vi "Three devices.vi"() -> ()   [LabVIEW 2015]
doc: "This example VI shows how to convert string data elements to numeric elements so it can be graphed and displayed on an XY Graph."
uses:
  <instrlib>/Keithley 27XX/Public/Configure/Measurement Specific/Configure Thermocouple.vi
  <instrlib>/Ke24xx/Ke24xx.llb/Ke24xx Configure Source Volt/Cur Level.vi
  <instrlib>/Ke24xx/Ke24xx.llb/Ke24xx Enable/Disable Source Output.vi
  <instrlib>/Keithley 27XX/Keithley 27XX.lvlib
panel:
  in  "Compliance":dbl=1.0 min=-1100.0 max=1100.0 step=1.0 format="%.2p"
  out "error out Cryocon":errorcluster
  out "error out 2425":errorcluster
  in  "Loop 2":bool
  in  "level":dbl=12.0 min=-1100.0 max=1100.0 step=1.0 format="%.2p"
  in  "range":i32
  in  "function":i32(slide)
  in  "error in (no error) 2":errorcluster
  in  "reset device":u16(slide)=1
  in  "id query":u16(slide)=1
  in  "resource name":string="GPIB0::20::INSTR"
  out "Delta":dbl
  out "Variance":string
  in  "Setpoint":dbl=300.0
  in  "D":sgl format="%.2f"
  in  "I":sgl=30.0 min=0 step=1 format="%.2f"
  in  "P":sgl=5.0 format="%.2f"
  in  "Output":u8(ring) items=["Loop 1", "Loop 2"]
  in  "Loop 1":bool
  out "Minimum":string
  out "Time Since Reset (Mins)":string
  out "Maximum":string
  out "Offset":string
  out "Cryocon Temp":dbl(graph)
  in  "Set Input":u8(ring) items=["ChA", "ChB", "ChC", "ChD"]
  in  "error in (no error)":errorcluster
  in  "baud rate (9600)":u32=9600
  in  "Port":string="10::INSTR"
  in  "Interface":u16(ring) items=["GPIB", "Serial"]
  in  "Save File?":bool
  out "Channel 3":dbl[](graph)
  out "Channel 2":dbl[](graph)
  out "Channel 1":dbl[](graph)
  in  "Enable Open Detector? (False)":bool
  in  "Simulated Reference Temperature (23 deg C)":dbl=23.0
  in  "Reference Junction Type (0: Simulated)":u16(ring)=1 items=["Simulated", "Internal", "External"]
  in  "Thermocouple Type (1: K)":u16(ring)=1 items=["J", "K", "T", "E", "R", "S", "B", "N"]
  in  "Column headers":string[](array[string])=["Time/s", "Cryocon Temp/C", "Ch101 Temp/C", "", "", "", ""]
  in  "Number of channels":i32=1
  in  "Pause/Continue":bool
  in  "stop":bool
  out "Iterations":i32
  out "concatenated string":string
  in  "file (use dialog)":path=path "C:/Users/Guest_2/Desktop/Zong Long/Data trial.txt"
  in  "Function (6: Temp)":u16(ring)=6 items=["DC Voltage", "AC Voltage", "DC Current", "AC Current", "Resistance", "Four-Wire Resistance", "Temperature (C)", "Frequency", "Period", "Continuity"]
  in  "Channel List (101)":string="101"
  in  "Serial Configuration":T1={"Baud Rate (9600)"=9600, "Flow Control (1: XON/XOFF)"=1, "Termination Char (0:CR)"=0} {"Termination Char (0:CR)" items=["CR", "LF", "CRLF (Do not use)", "LFCR (Do not use)"]; "Flow Control (1: XON/XOFF)" items=["None", "XON/XOFF", "RTS/CTS (2701 Only)", "XON/XOFF & RTS/CTS (2701 Only)"]; "Baud Rate (9600)" items=["300"=300, "600"=600, "1200"=1200, "2400"=2400, "4800"=4800, "9600"=9600, "19.2k"=19200, "38.4k (2701 Only)"=38400, "57.6k (2701 Only)"=57600, "115.2k (2701 Only)"=115200]}
  in  "Keithley VISA \nresource name":refnum<visa-resource-name>="GPIB0::19::INSTR"
  # "Keithley 2425 INIT"
  # "Cryocon INIT"
  # "File INIT"
  # "Keithley 2700 INIT"
  # "Operations"
  # "Data"
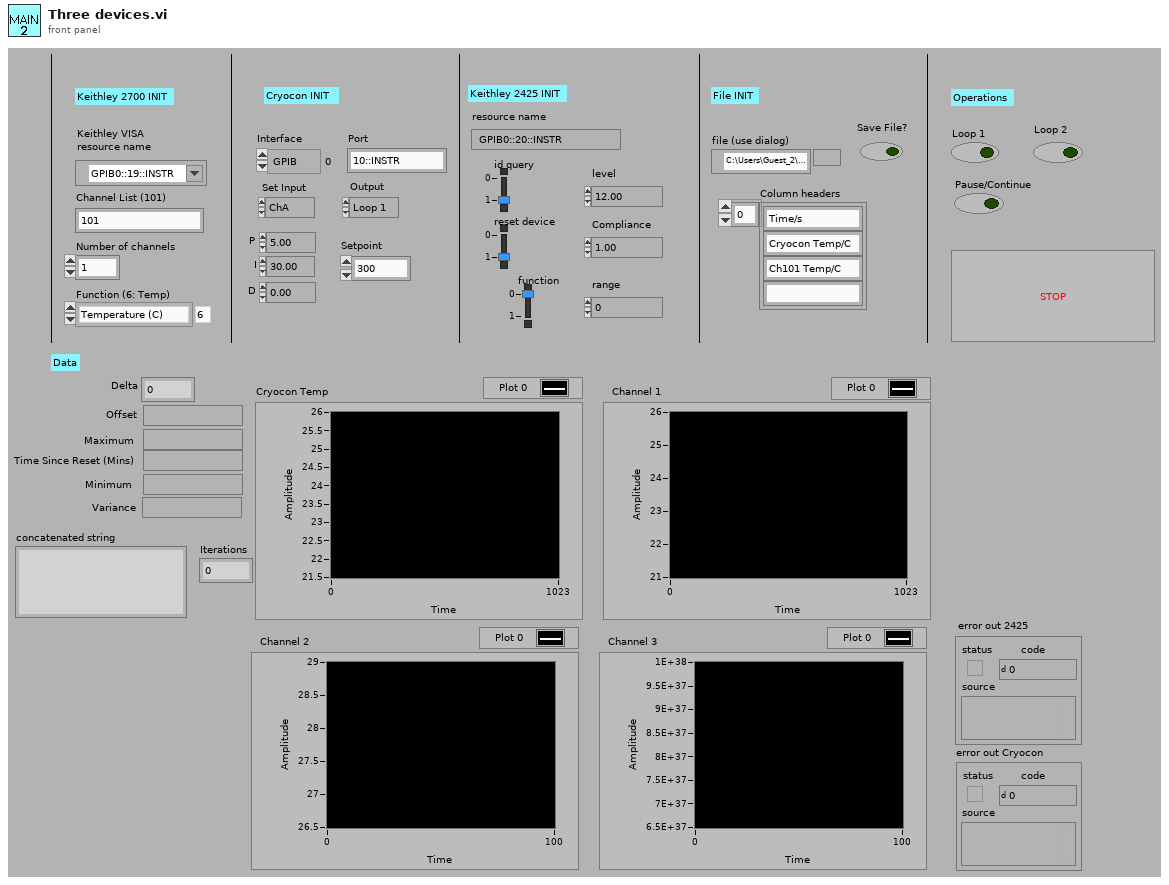
[diagram p1: front panel]
types:
  T1 = cluster{"Baud Rate (9600)":u32, "Flow Control (1: XON/XOFF)":u16, "Termination Char (0:CR)":u16}
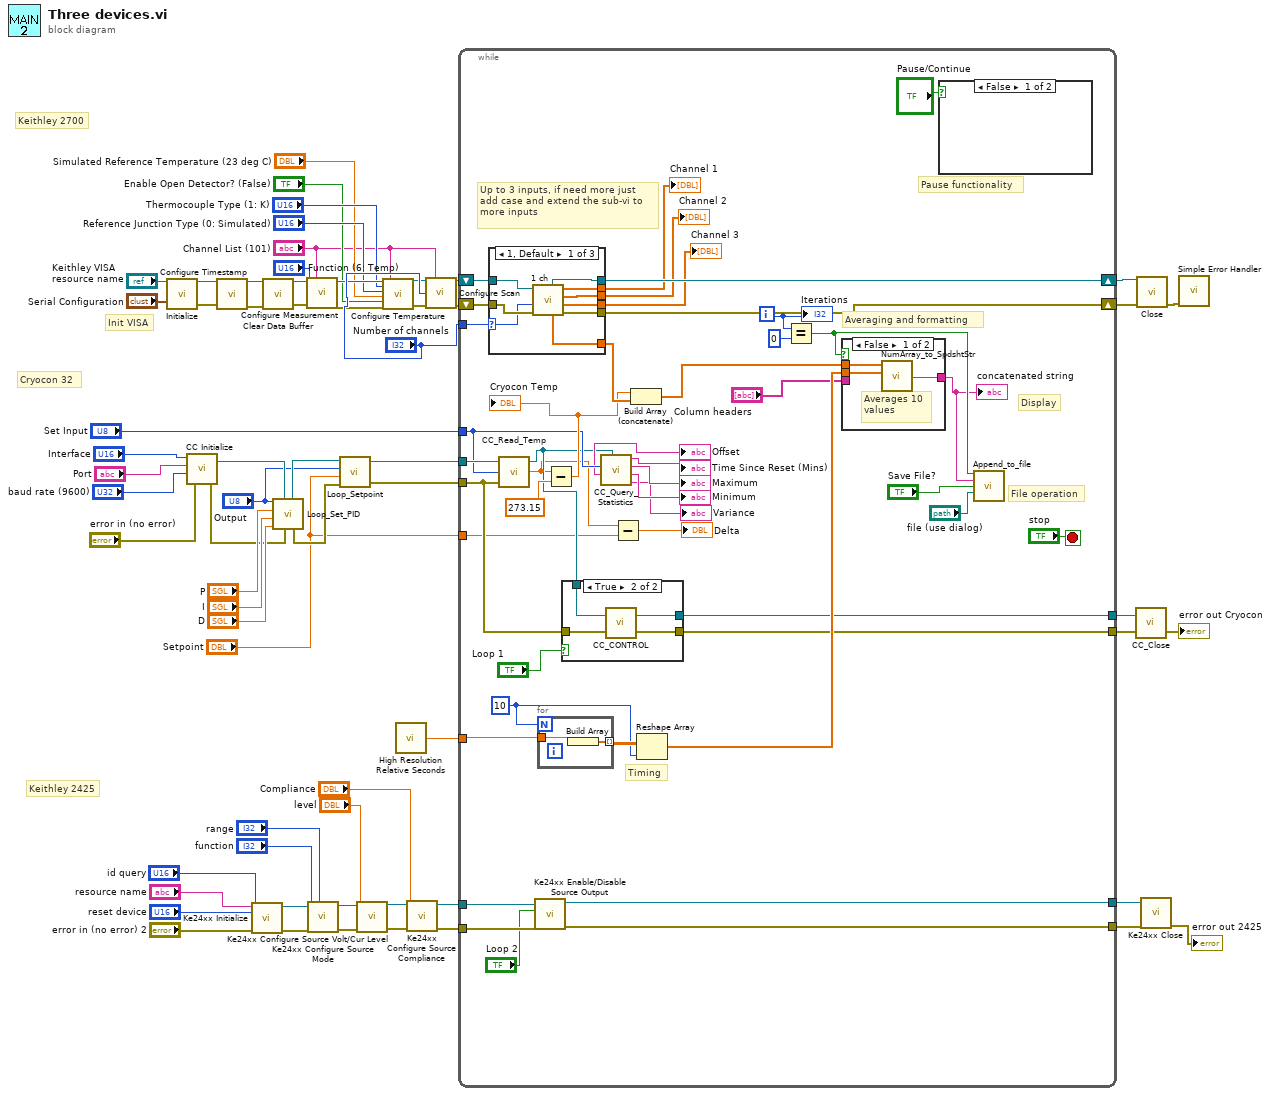
[diagram p0: block diagram]
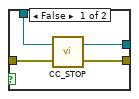
[diagram p2: hidden frame]
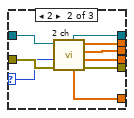
[diagram p3: hidden frame]
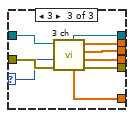
[diagram p4: hidden frame]
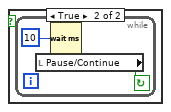
[diagram p5: hidden frame]
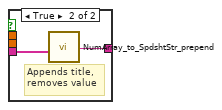
[diagram p6: hidden frame]
diagram:
  # "Keithley 2425"
  # "Cryocon 32"
  # "Keithley 2700"
  # "Init VISA"
  n1 = call <instrlib>:"Initialize.vi"("VISA resource name"="Keithley VISA \nresource name", "Serial Configuration"="Serial Configuration") -> ("VISA resource name out"=w60:refnum<visa-resource-name>, "error out"=w59:errorcluster)  [unwired: 12 in]
  n2 = call "CC Initialize.vi"("error in (no error)"="error in (no error)", "baud rate (9600)"="baud rate (9600)", "Port"="Port", "Interface"="Interface") -> ("error out"=w28:errorcluster, "VISA out"=w27:refnum<visa-resource-name>)
  n3 = call <instrlib>:"Configure Timestamp.vi"("VISA resource name"=w60, "error in (no error)"=w59) -> ("VISA resource name out"=w55:refnum<visa-resource-name>, "error out"=w54:errorcluster)  [unwired: 12 in]
  n4 = call <instrlib>:"Ke24xx Initialize.vi"("error in (no error)"="error in (no error) 2", "reset device"="reset device", "id query"="id query", "resource name"="resource name") -> ("error out"=w15:errorcluster, "instrument handle out"=w16:refnum<visa-resource-name>)  [unwired: 5 in, 1 out]
  n5 = call <instrlib>:"Clear Data Buffer.vi"("VISA resource name"=w55, "error in (no error)"=w54) -> ("VISA resource name out"=w53:refnum<visa-resource-name>, "error out"=w56:errorcluster)  [unwired: 12 in]
  n6 = call "Loop_Set_PID"("error in (no error)"=w28, "VISA In"=w27, "D"="D", "I"="I", "P"="P", "Output"="Output") -> ("error out"=w26:errorcluster, "VISA Out"=w25:refnum<visa-resource-name>)  [unwired: 4 in]
  n7 = call <instrlib>:"Configure Measurement.vi"("VISA resource name"=w53, "Scan List (Empty)"="Channel List (101)", "Function (0: DC Voltage)"="Function (6: Temp)", "error in (no error)"=w56) -> ("VISA resource name out"=w47:refnum<visa-resource-name>, "error out"=w44:errorcluster)  [unwired: 10 in]
  n8 = call <instrlib>:"Ke24xx Configure Source Mode.vi"("range"="range", "error in (no error)"=w15, "function"="function", "instrument handle"=w16) -> ("error out"=w11:errorcluster, "instrument handle out"=w12:refnum<visa-resource-name>)  [unwired: 5 in, 1 out]
  n9 = call "Loop_Setpoint.vi"("VISA in"=w25, "Loop"="Output", "Setpoint"="Setpoint", "error in"=w26) -> ("VISA out"=w24:refnum<visa-resource-name>, "ErrorOut"=w22:errorcluster)  [unwired: 1 in, 1 out]
  n10 = call "Ke24xx Configure Source Volt/Cur Level.vi"("error in (no error)"=w11, "level"="level", "instrument handle"=w12) -> ("error out"=w10:errorcluster, "instrument handle out"=w9:refnum<visa-resource-name>)  [unwired: 6 in, 1 out]
  n11 = call-poly <instrlib>:"Configure Temperature.vi"("VISA resource name"=w47, "Thermocouple Type (1: K)"="Thermocouple Type (1: K)", "Reference Junction Type (0: Simulated)"="Reference Junction Type (0: Simulated)", "Simulated Reference Temperature (23 deg C)"="Simulated Reference Temperature (23 deg C)", "Enable Open Detector? (False)"="Enable Open Detector? (False)", "error in (no error)"=w44, "Scan List (Empty)"="Channel List (101)") -> ("VISA resource name out"=w46:refnum<visa-resource-name>, "error out"=w45:errorcluster)  [unwired: 11 in]
  n12 = call <vilib>:"High Resolution Relative Seconds.vi"() -> ("relative seconds"=w49:dbl)
  n13 = call <instrlib>:"Ke24xx Configure Source Compliance.vi"("error in (no error)"=w10, "level"="Compliance", "instrument handle"=w9) -> ("error out"=w6:errorcluster, "instrument handle out"=w7:refnum<visa-resource-name>)  [unwired: 6 in, 1 out]
  n14 = call <instrlib>:"Configure Scan.vi"("VISA resource name"=w46, "Channel List (101:110)"="Channel List (101)", "Sample Count (100)"="Number of channels", "error in (no error)"=w45) -> ("VISA resource name out"=w51:refnum<visa-resource-name>, "error out"=w50:errorcluster)  [unwired: 10 in]
  n15 = while {
    shift-right: [w107] -> w57
    shift-left: w51 -> [w106]
    shift-right: [w108] -> w58
    shift-left: w50 -> [w105]
    tunnel: w49 -> [w103]
    tunnel: "Number of channels" -> [w96]
    tunnel: "Set Input" -> [w82]
    tunnel: w24 -> [w87]
    tunnel: w22 -> [w75]
    tunnel: [w74] -> w33
    tunnel: [w73] -> w32
    tunnel: "Setpoint" -> [w70]
    tunnel: w7 -> [w68]
    tunnel: w6 -> [w67]
    tunnel: [w65] -> w5
    tunnel: [w64] -> w4
    i -> [w98]
    stop <- "stop" stop-if-true
    w95 = 10 ("x")
    # "Timing"
    # "Up to 3 inputs, if need more just\nadd case and extend the sub-vi to\nmore inputs"
    # "Display"
    # "Averaging and formatting"
    # "File operation"
    # "Pause functionality"
    n16 = case shown="1, Default" w96 {
      selector: w96 -> [w124 w131 w140]
      tunnel: [w120 w132 w141] -> w108
      tunnel: [w122 w129 w139] -> w107
      tunnel: w106 -> [w123 w134 w142]
      tunnel: w105 -> [w125 w133 w143]
      tunnel: [w119 w127 w137] -> w92
      tunnel: [w118 w128 w136] -> w94
      tunnel: [w117 w130 w135] -> w93
      tunnel: [w121 w126 w138] -> w85
      frame 1, Default {
        n17 = call "1 ch.vi"("error out"=w125, "Number of channels"=w124, "VISA resource name out"=w123) -> ("error out 2"=w120:errorcluster, "output array 3"=w117:dbl[], "output array 2"=w118:dbl[], "Means of 10"=w119:dbl[], "output array"=w121:dbl[], "VISA resource name out 2"=w122:refnum<visa-resource-name>)  [unwired: 3 in]
      }
      frame 2 {
        n18 = call "2 ch.vi"("error out"=w133, "Number of channels"=w131, "VISA resource name out"=w134) -> ("error out 2"=w132:errorcluster, "Means of 12"=w130:dbl[], "Means of 11"=w128:dbl[], "Means of 10"=w127:dbl[], "output array"=w126:dbl[], "VISA resource name out 2"=w129:refnum<visa-resource-name>)  [unwired: 3 in]
      }
      frame 3 {
        n19 = call "3 ch.vi"("error out"=w143, "Number of channels"=w140, "VISA resource name out"=w142) -> ("error out 2"=w141:errorcluster, "Means of 12"=w135:dbl[], "Means of 11"=w136:dbl[], "Means of 10"=w137:dbl[], "output array"=w138:dbl[], "VISA resource name out 2"=w139:refnum<visa-resource-name>)  [unwired: 3 in]
      }
    }
    "Channel 3" <- w93
    "Channel 2" <- w94
    "Channel 1" <- w92
    n20 = call "CC_Read_Temp.vi"("error in (no error)"=w75, "Input"=w82, "VISA In"=w87) -> ("Temperature"=w71:dbl, "VISA Out"=w76:refnum<visa-resource-name>)  [unwired: 1 out]
    n21 = call "Ke24xx Enable/Disable Source Output.vi"("error in (no error)"=w67, "state"="Loop 2", "instrument handle"=w68) -> ("error out"=w64:errorcluster, "instrument handle out"=w65:refnum<visa-resource-name>)  [unwired: 6 in, 1 out]
    n22 = for {
      N: w95 -> [_]
      tunnel: w103 -> [w147]
      tunnel: [w146] -> w102 mode=indexing
      n23 = Build Array(w147) -> (w146:dbl[])
    }
    n24 = Subtract(x=w71, y=273.15) -> (x-y=w83:dbl)
    "Cryocon Temp" <- w83
    n25 = case shown="True" "Loop 1" {
      tunnel: w76 -> [w112 w116]
      tunnel: w75 -> [w111 w115]
      tunnel: [w110 w114] -> w74
      tunnel: [w109 w113] -> w73
      frame False {
        n26 = call "CC_STOP.vi"("error in (no error)"=w111, "VISA In"=w112) -> ("error out"=w109:errorcluster, "VISA Out"=w110:refnum<visa-resource-name>)
      }
      frame True {
        n27 = call "CC_CONTROL.vi"("error in (no error)"=w115, "VISA In"=w116) -> ("error out"=w113:errorcluster, "VISA Out"=w114:refnum<visa-resource-name>)
      }
    }
    n28 = call "CC_Query_Statistics.vi"("VISA In"=w76, "Input"=w82) -> ("Variance"=→"Variance":string, "Minimum"=→"Minimum":string, "Maximum"=→"Maximum":string, "Time Since Reset"=→"Time Since Reset (Mins)":string, "Offset"=→"Offset":string)  [unwired: 2 in, 3 out]
    n29 = Subtract(x=w71, y=w70) -> (x-y=→"Delta":dbl)
    n30 = Build Array (concatenate)(w83, w85) -> (w86:dbl[])
    n31 = Reshape Array(w102, w95) -> (w101:dbl[])
    n32 = Equal?(x=w98, y=0) -> (x = y?=w90:bool)
    n33 = case shown="False" w90 {
      tunnel: w86 -> [w150 _]
      tunnel: w101 -> [w149 _]
      tunnel: [w148 w152] -> w89
      tunnel: "Column headers" -> [_ w151]
      frame False {
        # "Averages 10 \nvalues"
        n34 = call "NumArray_to_SpdshtStr.vi"("element 2"=w149, "element"=w150) -> ("concatenated string"=w148:string)  [unwired: 8 in, 1 out]
      }
      frame True {
        # "Appends title,\nremoves value"
        n35 = call "NumArray_to_SpdshtStr_prepend.vi"("Column headers"=w151) -> ("concatenated string"=w152:string)  [unwired: 10 in]
      }
    }
    "concatenated string" <- w89
    n36 = case shown="False" "Pause/Continue" {
      frame False {
      }
      frame True {
        n37 = while {
          stop <- w145 continue-if-true
          n38 = local read "Pause/Continue"() -> (w145:bool)
          n39 = Wait (ms)(milliseconds to wait=u32 10) -> ()  [unwired: 1 out]
        }
      }
    }
    n40 = call "Append_to_file.vi"("Boolean"=w90, "text"=w89, "Save File?"="Save File?", "file path (use dialog)"="file (use dialog)") -> ()  [unwired: 11 in, 1 out]
    "Iterations" <- w98
  }
  n41 = call "CC_Close.vi"("error in (no error)"=w32, "VISA In"=w33) -> ("error out"=→"error out Cryocon":errorcluster)  [unwired: 1 in]
  n42 = call <instrlib>:"Close.vi"("VISA resource name"=w57, "error in (no error)"=w58) -> ("error out"=w61:errorcluster)  [unwired: 13 in]
  n43 = call <instrlib>:"Ke24xx Close.vi"("error in (no error)"=w4, "instrument handle"=w5) -> ("error out"=→"error out 2425":errorcluster)  [unwired: 8 in, 1 out]
  n44 = call <vilib>:"Simple Error Handler.vi"("error in (no error)"=w61) -> ()  [unwired: 4 in, 5 out]
